vi "rohit1-d.vi"() -> ()   [LabVIEW 2009]
panel:
  in  "size":i32
  out "Array":dbl[](array[numeric])
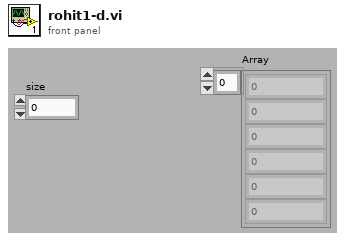
[diagram p1: front panel]
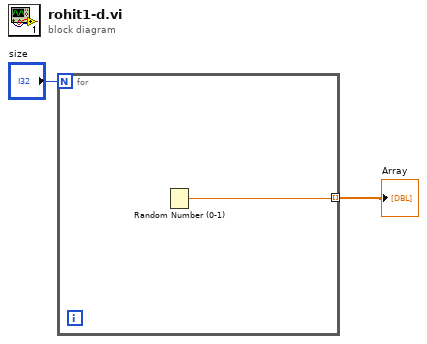
[diagram p0: block diagram]
diagram:
  n1 = for {
    N: "size" -> [_]
    tunnel: [w3] -> w2 mode=indexing
    n2 = Random Number (0-1)() -> (number: 0 to 1=w3:dbl)
  }
  "Array" <- w2
